vi "exec.vi"(8 "error in (no error)":errorcluster, 10 "context":refnum<class "Context.lvclass">, 11 "StopTest in":refnum<class "StopTest.lvclass">) -> (0 "error out":errorcluster, 2 "context 2":refnum<class "Context.lvclass">, 3 "StopTest out":refnum<class "StopTest.lvclass">)   [LabVIEW 2015, in "StopTest.lvclass"]
uses:
  StopTest.lvclass
  Context/Context.lvclass
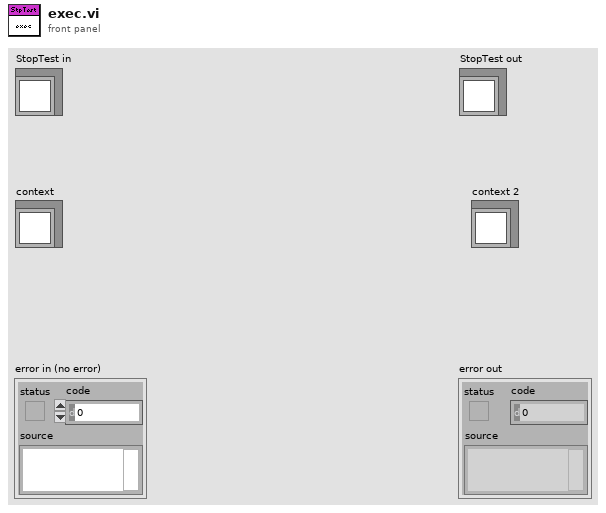
[diagram p1: front panel]
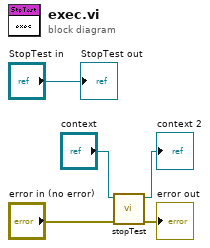
[diagram p0: block diagram]
diagram:
  n1 = call "stopTest.vi"("error in (no error)"="error in (no error)", "Context in"="context") -> ("error out"=→"error out":errorcluster, "Context out"=→"context 2":refnum<class "Context.lvclass">)  [unwired: 8 in]
  "StopTest out" <- "StopTest in"
